vi "Create Default Attributes.vi"(5 "Unique ID":string, 7 "Process Executive Ref":refnum<data-value>, 11 "Stop Bug Remover in":refnum<class "Stop Bug Remover.lvclass">) -> (3 "Stop Bug Remover out":refnum<class "Stop Bug Remover.lvclass">)   [LabVIEW 2019, in "Stop Bug Remover.lvclass"]
uses:
  <vilib>/gpm_packages/@cs/Car-wash/Source/Process Steps/Stop Bug Remover/Stop Bug Remover.lvclass
  <vilib>/gpm_packages/@cs/test-executive/Source/Test Executive/ITestExecutive/ITest Executive.lvclass
  478ab49c-73c8-47c5-8c9d-7d1b3c9be739.vi
  <vilib>/Utility/error.llb/Error Cluster From Error Code.vi
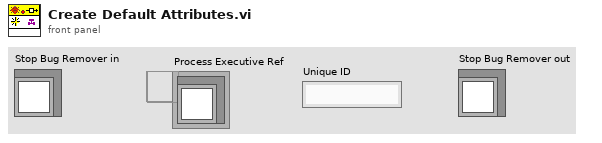
[diagram p1: front panel]
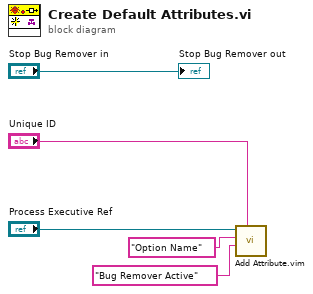
[diagram p0: block diagram]
diagram:
  n1 = call "Add Attribute.vim"("ID"="Unique ID", "Attribute"="Bug Remover Active" ("Item Name"), "Attribute Name"="Option Name" ("Item Name"), "Test Executive Ref"="Process Executive Ref") -> ()  [unwired: 4 in, 4 out]
  "Stop Bug Remover out" <- "Stop Bug Remover in"
